vi "getRef.vi"(8 "error in (no error)":errorcluster) -> (0 "error out":errorcluster, 2 "File Controller.lvclass":refnum<class "File Controller.lvclass">)   [LabVIEW 2015, in "File Controller.lvclass"]
uses:
  File Controller.lvclass
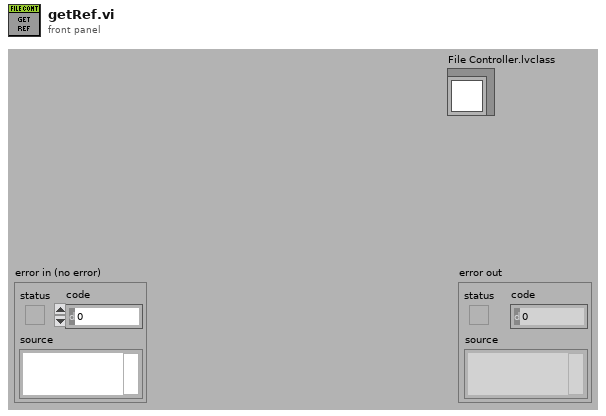
[diagram p1: front panel]
types:
  T1 = typedef "File Controller.lvclass/ClassAttributesRef.ctl" = refnum<data-value>
  T2 = typedef "File Controller.lvclass/ClassAttributes.ctl" = cluster{"Dummy":bool, "File Controller.lvclass":refnum<class "File Controller.lvclass">}
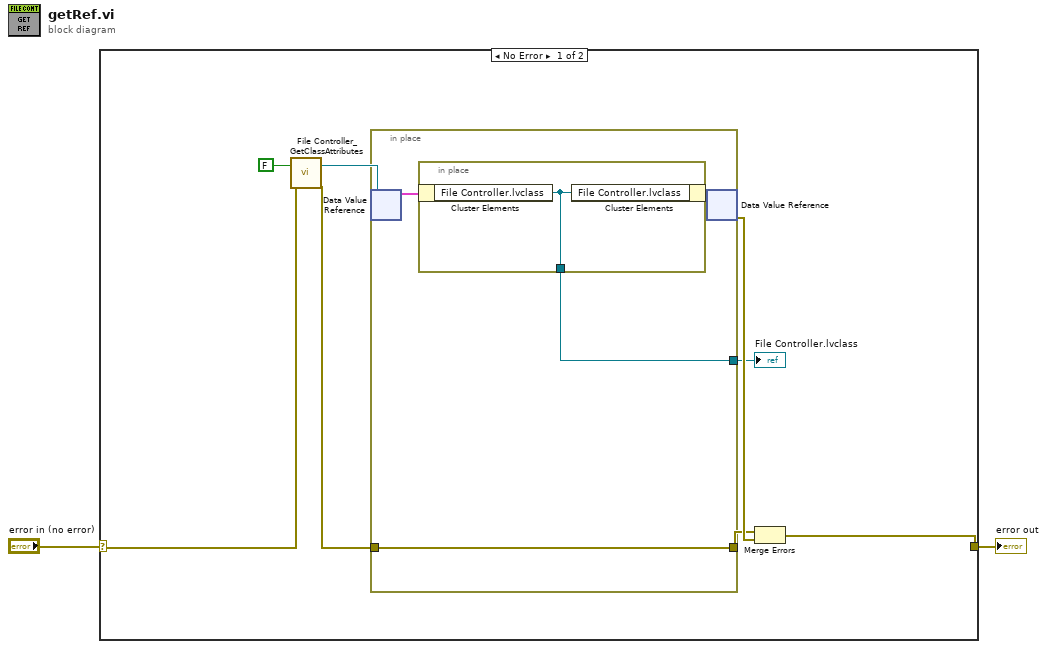
[diagram p0: block diagram]
diagram:
  n1 = case shown="No Error" "error in (no error)" {
    selector: "error in (no error)" -> [w7 w16]
    tunnel: [w10 w16] -> w1
    frame No Error {
      n2 = call "File Controller_GetClassAttributes.vi"("return data? (T)"=FALSE, "error in (no error)"=w7) -> ("class attributes ref"=w5:T1, "error out"=w6:errorcluster)  [unwired: 14 in, 2 out]
      n3 = in-place {
        in-place-border: w6 -> [w12]
        in-place-border: [w12] -> w8
        in-place-border: [w11] -> w4
        n4 = in-place-dvr #1(w5) -> (w13:T2)  [unwired: 1 out]
        n5 = in-place {
          in-place-border: [w15] -> w11
          n6 = in-place-cluster #2(w13) -> ("File Controller.lvclass"=w15:refnum<class "File Controller.lvclass">)
          n7 = in-place-cluster #2("File Controller.lvclass"=w15) -> (w14:T2)
        }
        n8 = in-place-dvr #1(w14) -> (w9:errorcluster)  [unwired: 1 out]
      }
      "File Controller.lvclass" <- w4
      n9 = Merge Errors(w8, w9) -> (w10:errorcluster)
    }
    frame Error {
    }
  }
  "error out" <- w1
